vi "Read Numeric as DBL.vi"(8 "error in (no error)":errorcluster, 10 "Tag":string, 11 "Var Bus in":refnum<class "Multi_Bus.lvclass">) -> (0 "error out":errorcluster, 2 "Numeric":dbl, 3 "Var Bus out":refnum<class "Multi_Bus.lvclass">)   [LabVIEW 2021, in "Multi_Bus.lvclass"]
uses:
  Multi_Bus.lvclass
  Multi_Bus.lvclass/Multi_Bus.ctl
  Properties/Read Var Map.vi
  Support/Incorrect Tag String Error.vi
  <vilib>/TSA/Abstract Data Classes/Abs_Types/Type/Abs_Type.lvclass
  <vilib>/TSA/Abstract Data Classes/Abs_Types/Numeric/Abs_Numeric.lvclass
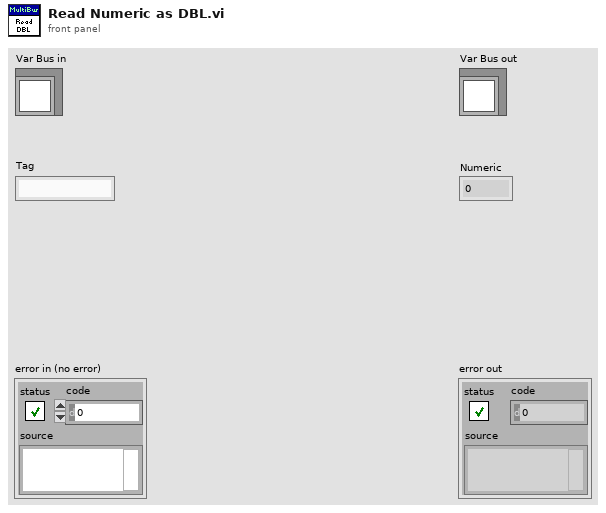
[diagram p1: front panel]
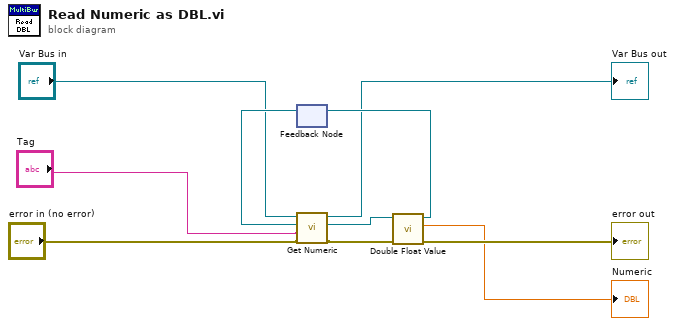
[diagram p0: block diagram]
diagram:
  n1 = feedback #1() -> (w3:refnum<class "Abs_Numeric.lvclass">)  [unwired: 1 in]
  n2 = call-dynamic "Get Numeric.vi"("error in (no error)"="error in (no error)", "Tag"="Tag", "Value Type"=w3, "Var Bus in"="Var Bus in") -> ("error out"=w7:errorcluster, "Value Out"=w6:refnum<class "Abs_Numeric.lvclass">, "Var Bus out"=→"Var Bus out":refnum<class "Multi_Bus.lvclass">)  [unwired: 5 in]
  n3 = call-dynamic "Double Float Value.vi"("error in (no error)"=w7, "Numeric in"=w6) -> ("error out"=→"error out":errorcluster, "Double"=→"Numeric":dbl, "Numeric out"=w8:refnum<class "Abs_Numeric.lvclass">)  [unwired: 7 in]
  n4 = feedback-in #1(w8) -> ()
